vi "getOffsetToUTC.vi"(11 "Epoch":refnum<class "Epoch.lvclass">) -> (2 "Offset to UTC":i64)   [LabVIEW 2018, in "Epoch.lvclass"]
uses:
  Epoch.lvclass
  <vilib>/Utility/miscctls.llb/LVDateTimeRec.ctl
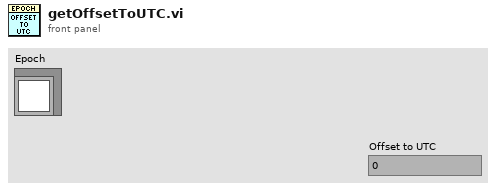
[diagram p1: front panel]
types:
  T1 = typedef "LVDateTimeRec.ctl" = cluster{"fractional second":dbl, "second":i32, "minute":i32, "hour":i32, "day of month":i32, "month":i32, "year":i32, "day of week":i32, "day of year":i32, "DST":i32}
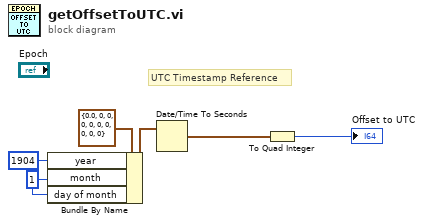
[diagram p0: block diagram]
diagram:
  w5 = 1 ("month")
  # "UTC Timestamp Reference"
  n1 = Bundle By Name(cluster=T1 {"fractional second"=0.0, "second"=0, "minute"=0, "hour"=0, "day of month"=0, "month"=0, "year"=0, "day of week"=0, "day of year"=0, "DST"=0} ("date time rec"), "year"=1904, "month"=w5, "day of month"=w5) -> (w3:T1)
  n2 = Date/Time To Seconds(2:w3) -> (0:w1:timestamp)  [unwired: 1 in]
  n3 = To Quad Integer(1:w1) -> (0:→"Offset to UTC":i64)
